vi "GDSString_ParseTextBasedCode.vi"(8 "error in (no error)":errorcluster, 11 "TextIn":string) -> (0 "error out":errorcluster, 3 "Classes":T1[](array[typedef]))   [LabVIEW 2012]
uses:
  <resource>/Framework/Providers/Open_GDS/ClassProviders/Common/String/GDSString_ClassDescriptionType.ctl
  <resource>/Framework/Providers/Open_GDS/ClassProviders/Common/String/GDSString_AccessScopeModifierType.ctl
  <resource>/Framework/Providers/Open_GDS/ClassProviders/Common/String/GDSString_ModifierType.ctl
  <resource>/Framework/Providers/Open_GDS/ClassProviders/Common/String/GDSString_MethodDescriptionType.ctl
  <resource>/Framework/Providers/Open_GDS/ClassProviders/Common/CommonVIs/CommonVIs_AttributeType.ctl
  <resource>/Framework/Providers/Open_GDS/ClassProviders/Common/CommonVIs/CommonVIs_AttributeDataType.ctl
  <resource>/Framework/Providers/Open_GDS/ClassProviders/Common/String/GDSString_ClassParentType.ctl
  <resource>/Framework/Providers/Open_GDS/ClassProviders/Common/String/GDSString_ClassType.ctl
  <resource>/Framework/Providers/Open_GDS/ClassProviders/Common/String/GDSString_ClassOwnerType.ctl
  <resource>/Framework/Providers/Open_GDS/ClassProviders/Common/CommonVIs/CommonVIs_EnumType.ctl
  <resource>/Framework/Providers/Open_GDS/ClassProviders/Common/CommonVIs/CommonVIs_StructType.ctl
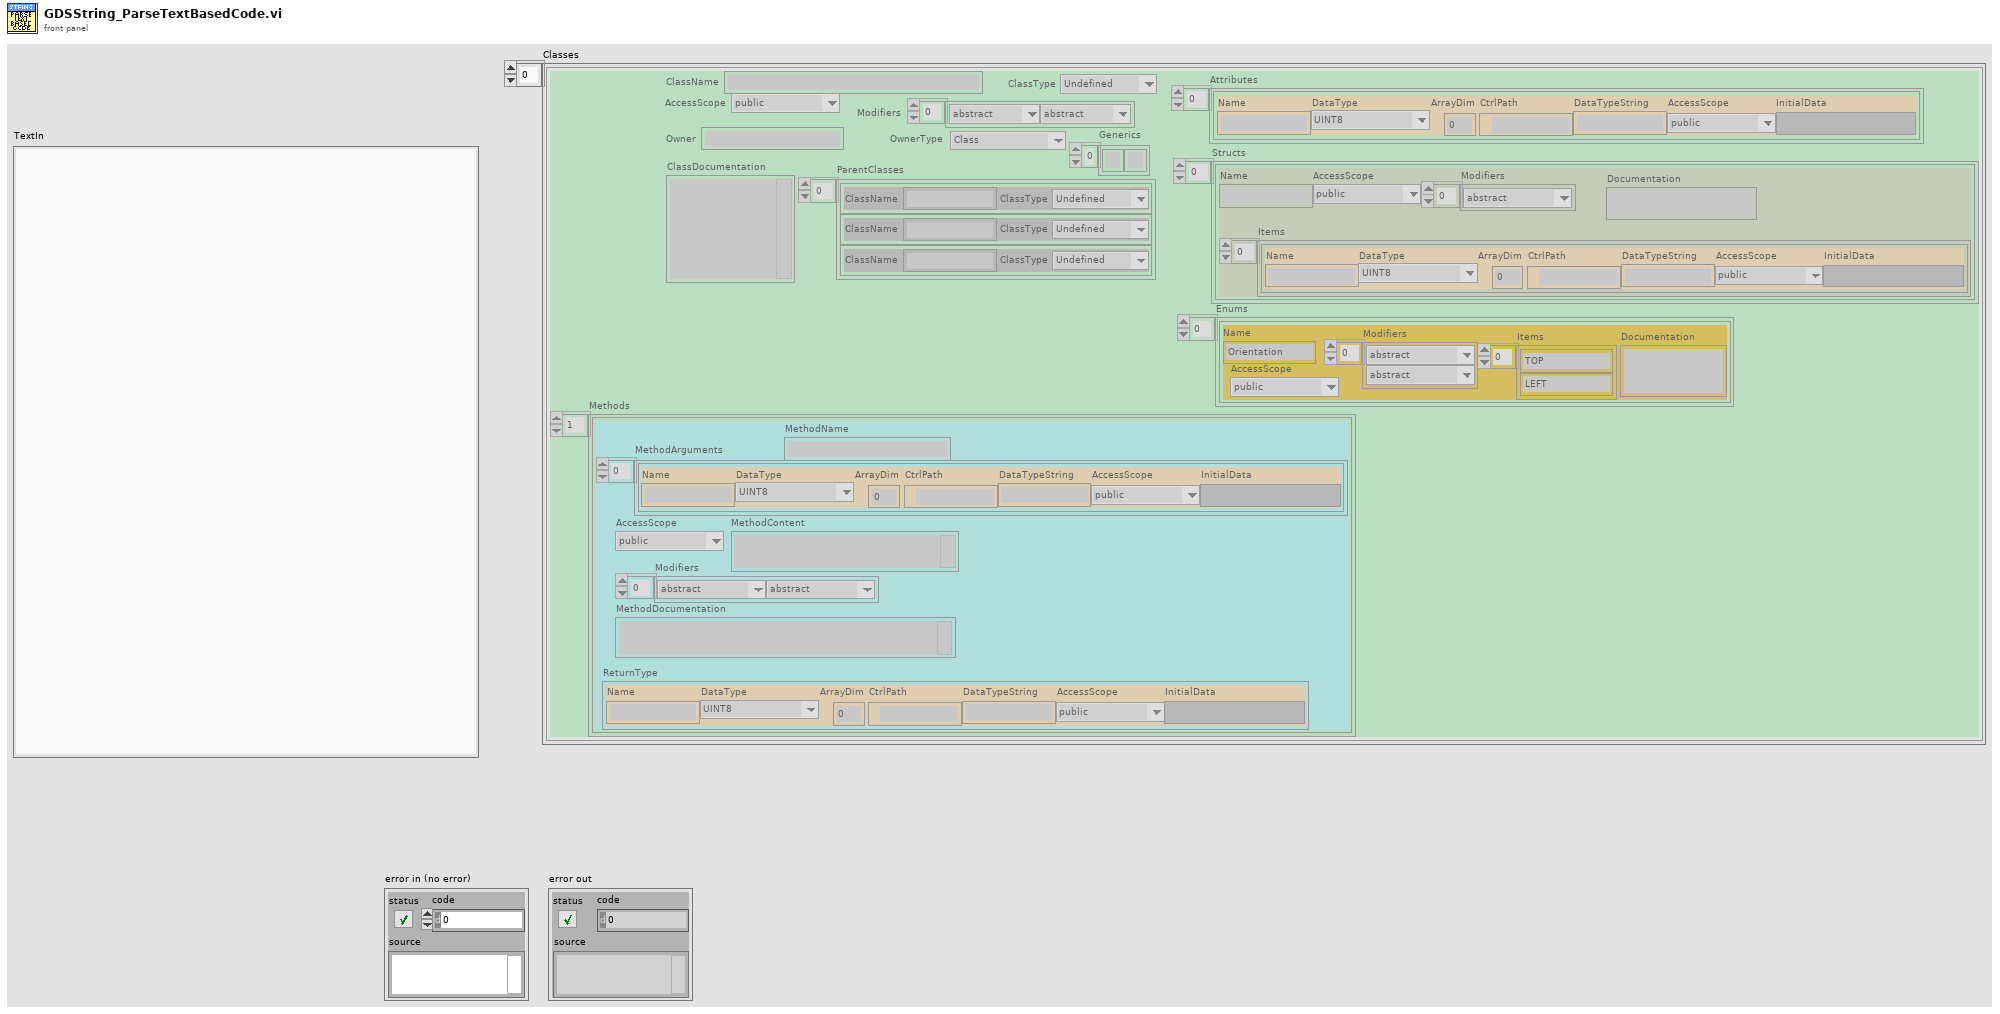
[diagram p1: front panel]
types:
  T1 = typedef "GDSString_ClassDescriptionType.ctl" = cluster{"ClassName":string, "AccessScope":T2, "Modifiers":T3[], "ClassDocumentation":string, "Methods":T4[], "ParentClasses":T7[], "ClassType":T8, "Owner":string, "OwnerType":T9, "Generics":string[], "Attributes":T5[], "Enums":T10[], "Structs":T11[]}
  T2 = typedef "GDSString_AccessScopeModifierType.ctl" = enum16{"public", "private", "protected", "internal"}
  T3 = typedef "GDSString_ModifierType.ctl" = enum16{"abstract", "static", "final", "synchronized", "strictfp", "async", "const", "event", "extern", "new", "override", "partial", "readonly", "sealed", "unsafe", "virtual", "volatile"}
  T4 = typedef "GDSString_MethodDescriptionType.ctl" = cluster{"ReturnType":T5, "MethodName":string, "AccessScope":T2, "Modifiers":T3[], "MethodDocumentation":string, "MethodContent":string, "MethodArguments":T5[]}
  T5 = typedef "CommonVIs_AttributeType.ctl" = cluster{"Name":string, "DataType":T6, "ArrayDim":i32, "CtrlPath":path, "DataTypeString":string, "AccessScope":T2, "InitialData":variant}
  T6 = typedef "CommonVIs_AttributeDataType.ctl" = enum16{"UINT8", "INT8", "UINT16", "INT16", "UINT32", "INT32", "UINT64", "INT64", "SGL", "DBL", "EXT", "CSG", "CDB", "CXT", "TimeStamp", "STRING", "PATH", "BOOL", "ENUM", "RefNum", "VIRefNum", "LabVIEW Class", "Cluster", "Variant", "TypeDef", "Waveform", "LabVIEW Object", "Other", "void"}
  T7 = typedef "GDSString_ClassParentType.ctl" = cluster{"ClassName":string, "ClassType":T8}
  T8 = typedef "GDSString_ClassType.ctl" = enum16{"Undefined", "Class", "Interface"}
  T9 = typedef "GDSString_ClassOwnerType.ctl" = enum16{"NoOwner", "Class", "Package/NameSpace"}
  T10 = typedef "CommonVIs_EnumType.ctl" = cluster{"Name":string, "AccessScope":T2, "Modifiers":T3[], "Items":string[], "Documentation":string}
  T11 = typedef "CommonVIs_StructType.ctl" = cluster{"Name":string, "AccessScope":T2, "Modifiers":T3[], "Items":T5[], "Documentation":string}
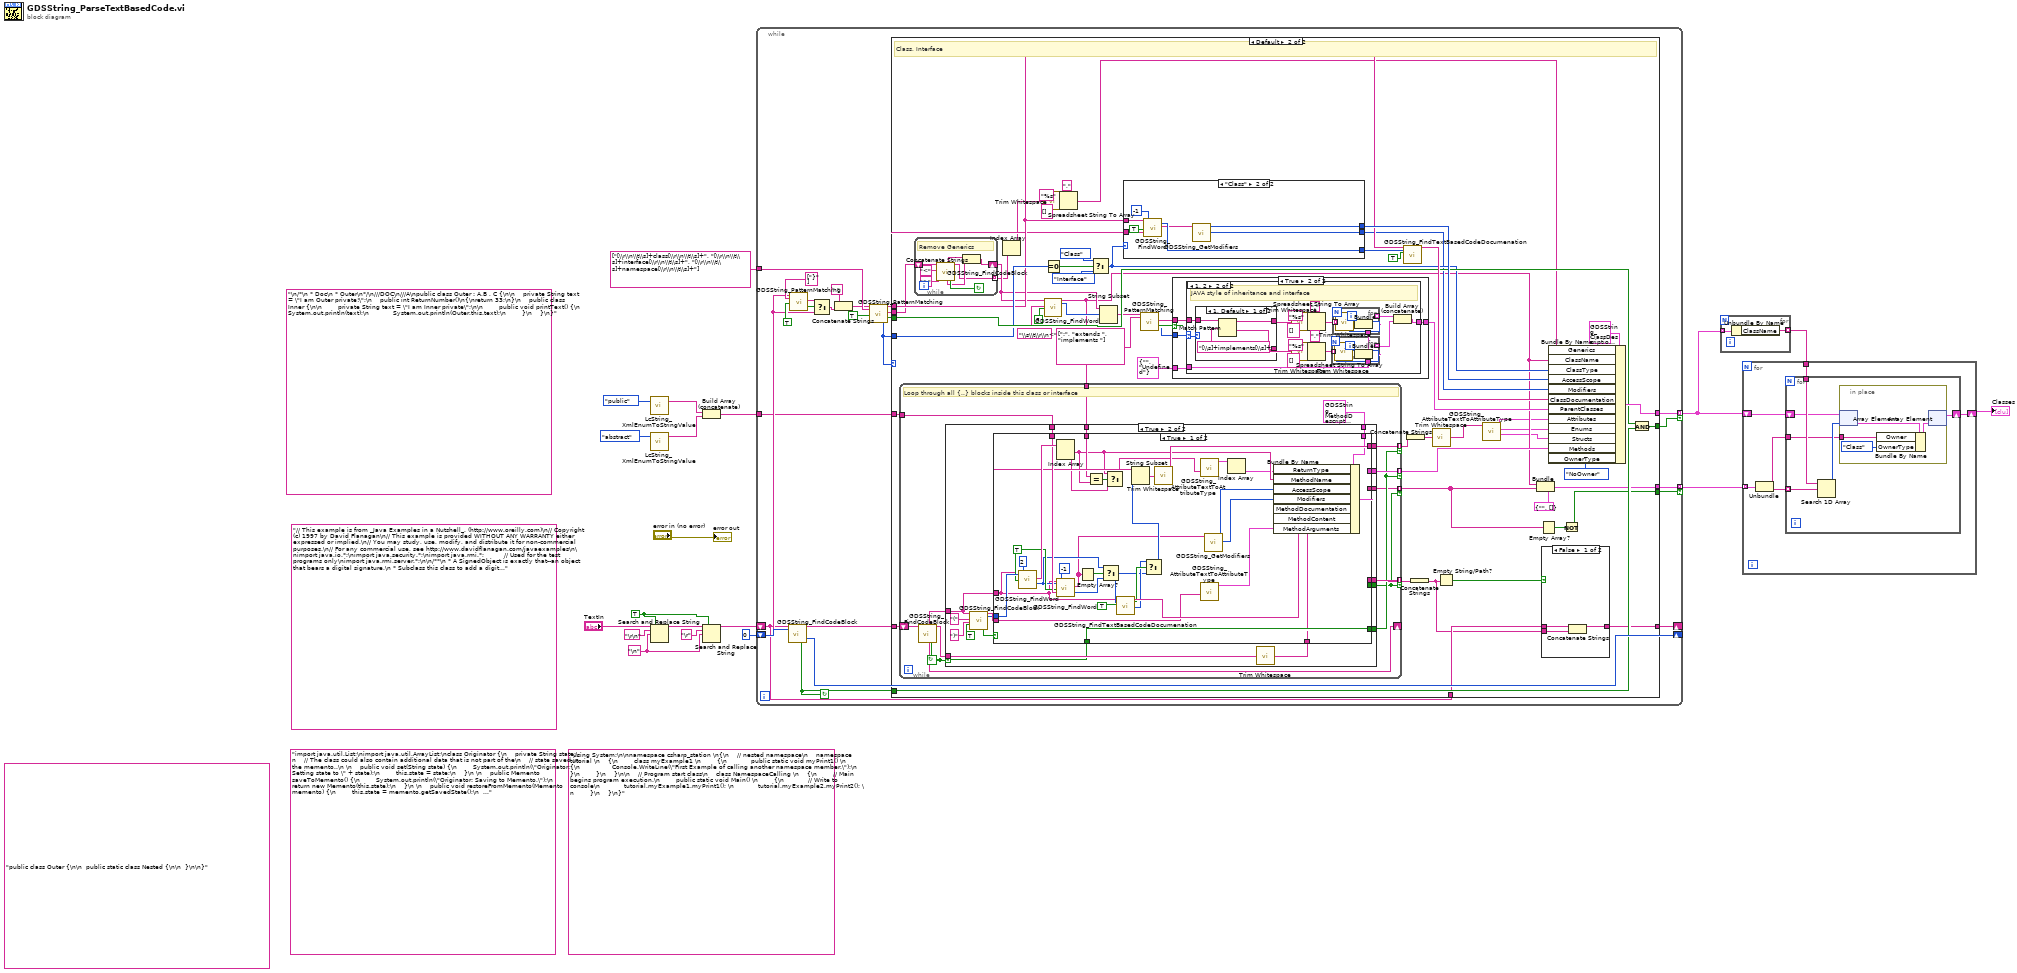
[diagram p0: block diagram]
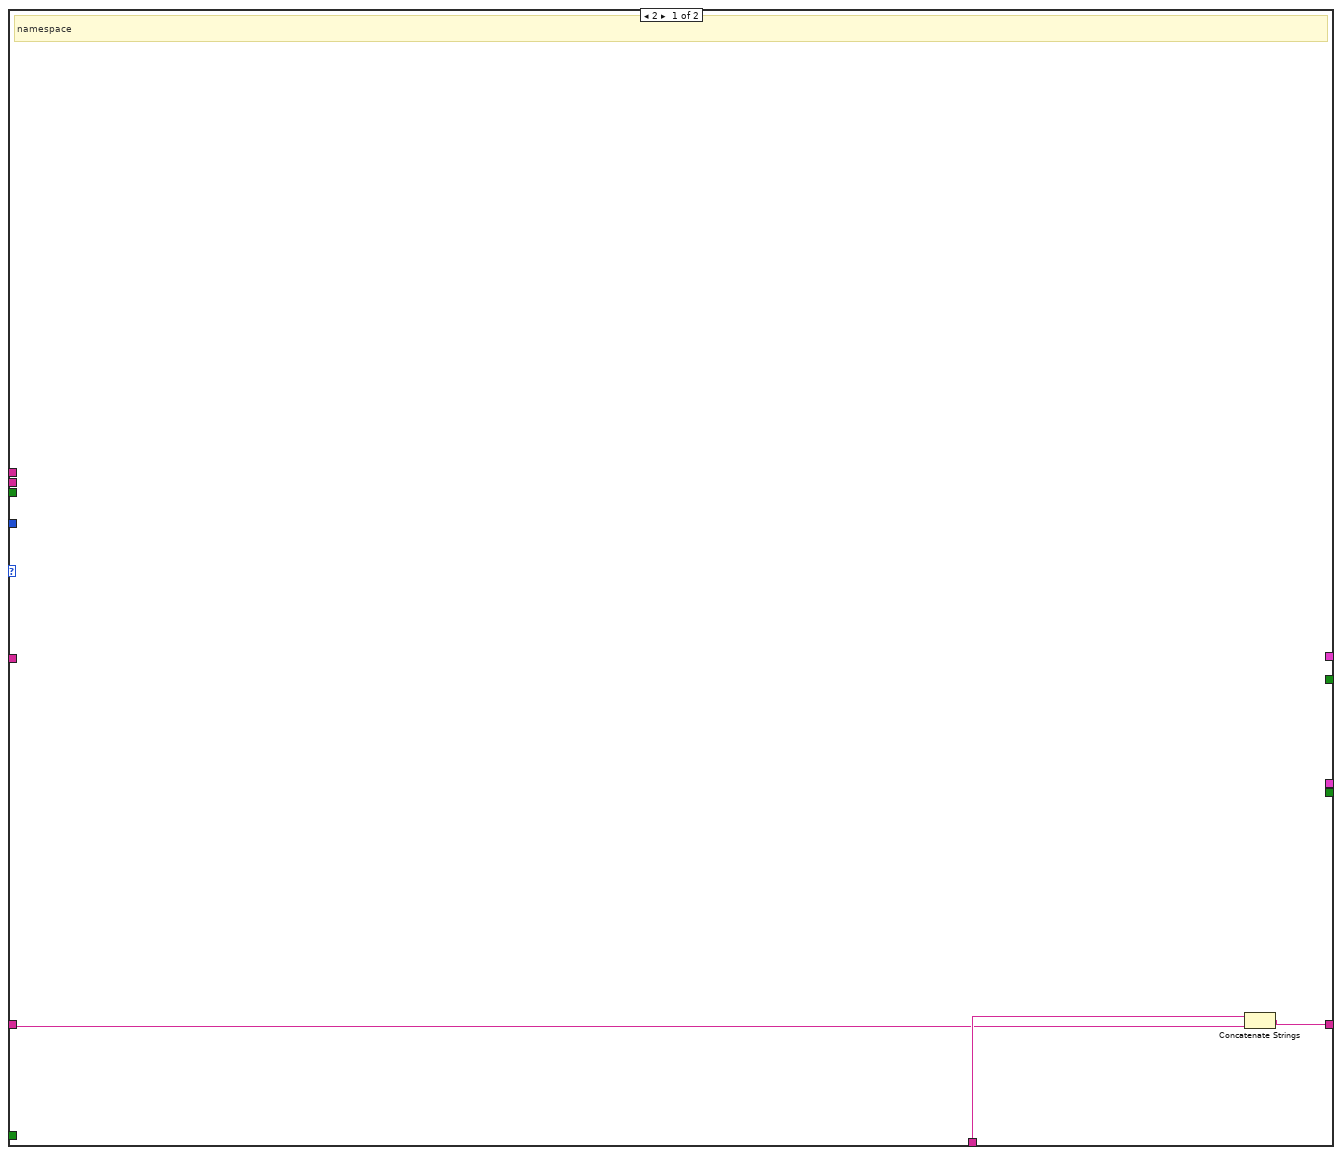
[diagram p2: hidden frame]
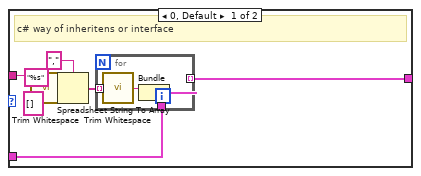
[diagram p5: hidden frame]
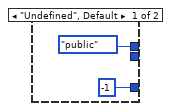
[diagram p7: hidden frame]
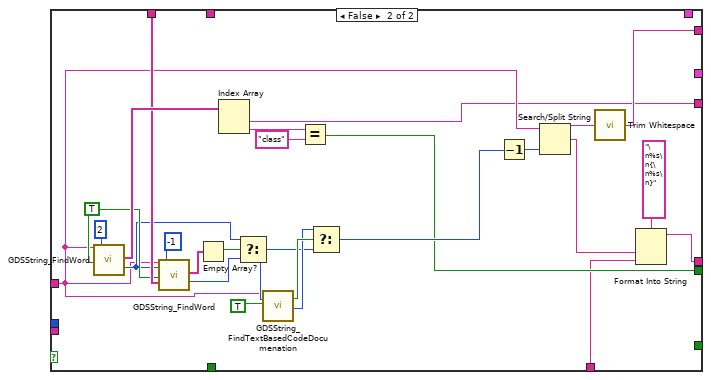
[diagram p9: hidden frame]
diagram:
  (unwired) "using System;\n\nnamespace csharp_station \n{\n    // nested namespace\n    namespace tutorial \n    {\n        class myExample1 \n        {\n            public static void myPrint1() \n            {\n                Console.WriteLine(\"First Example of calling another namespace member.\");\n            }\n        }\n    }\n\n    // Program start class\n    class NamespaceCalling \n    {\n        // Main begins program execution.\n        public static void Main() \n        {\n            // Write to console\n            tutorial.myExample1.myPrint1(); \n            tutorial.myExample2.myPrint2(); \n        }\n    }\n}" ("text")
  (unwired) "public class Outer {\n\n  public static class Nested {\n\n  }\n\n}" ("text")
  (unwired) "import java.util.List;\nimport java.util.ArrayList;\nclass Originator {\n    private String state;\n    // The class could also contain additional data that is not part of the\n    // state saved in the memento..\n \n    public void set(String state) {\n        System.out.println(\"Originator: Setting state to \" + state);\n        this.state = state;\n    }\n \n    public Memento saveToMemento() {\n        System.out.println(\"Originator: Saving to Memento.\");\n        return new Memento(this.state);\n    }\n \n    public void restoreFromMemento(Memento memento) {\n        this.state = memento.getSavedState();\n        System.out.println(\"Originator: State after restoring from Memento: \" + state);\n    }\n \n    public static class Memento {\n        private final String state;\n \n        public Memento(String stateToSave) {\n            state = stateToSave;\n        }\n \n        public String getSavedState() {\n            return state;\n        }\n    }\n}\n \nclass Caretaker {\n    public static void main(String[] args) {\n        List<Originator.Memento> savedStates = new ArrayList<Originator.Memento>();\n \n        Originator originator = new Originator();\n        originator.set(\"State1\");\n        originator.set(\"State2\");\n        savedStates.add(originator.saveToMemento());\n        originator.set(\"State3\");\n        // We can request multiple mementos, and choose which one to roll back to.\n        savedStates.add(originator.saveToMemento());\n        originator.set(\"State4\");\n \n        originator.restoreFromMemento(savedStates.get(1));   \n    }\n}" ("text")
  (unwired) "// This example is from _Java Examples in a Nutshell_. (http://www.oreilly.com)\n// Copyright (c) 1997 by David Flanagan\n// This example is provided WITHOUT ANY WARRANTY either expressed or implied.\n// You may study, use, modify, and distribute it for non-commercial purposes.\n// For any commercial use, see http://www.davidflanagan.com/javaexamples\n\nimport java.io.*;\nimport java.security.*;\nimport java.rmi.*;          // Used for the test programs only\nimport java.rmi.server.*;\n\n/**\n * A SignedObject is exactly that--an object that bears a digital signature.\n * Subclass this class to add a digital signature to any class you want.\n * Note, however, that the signature is computed using serialization, so only\n * the serializable, non-transient fields of a subclass are included in\n * the signature computation.\n **/\npublic class SignedObject implements Serializable {\n  protected String signername;               // Who is doing the signing\n  protected String algorithm;                // What algorithm to use.\n  private byte[] signature;                  // The bytes of the signature\n  transient private boolean signing = false; // A flag used below.\n\n  /**\n   * This method computes a digital signature for the current state of the\n   * object, excluding the signature-related state of this class.\n   * That is, the signature is based only on the state of the subclasses.\n   * The arguments specify who is signing the object, and what digital \n   * signature algorithm to use.\n   * \n   * Note that no other threads should be modifying the object while\n   * this computation is being performed.  If a subclass will be used in a \n   * multi-threaded environment, this means that methods of the subclass\n   * that modify its state should be synchronized like this one is.\n   **/\n  public synchronized void sign(String signername, String algorithm) \n       throws IOException, InvalidKeyException, \n         SignatureException, NoSuchAlgorithmException \n  {\n    // Save the arguments for use by verify()\n    this.signername = signername;\n    this.algorithm = algorithm;\n\n    // Get a Signature object to compute the signature with\n    Signature s = Signature.getInstance(algorithm);\n\n    // Get a Signer object representing the signer\n    Signer signer = \n      (Signer)IdentityScope.getSystemScope().getIdentity(signername);\n\n    // Initialize the Signature object using the PrivateKey of the Signer\n    s.initSign(signer.getPrivateKey());\n\n    // Create an ObjectOutputStream that writes its output to a \n    // ByteArrayStream.  This is how we capture the state of the object\n    // so that it can be signed.\n    ByteArrayOutputStream bout = new ByteArrayOutputStream();\n    ObjectOutputStream out = new ObjectOutputStream(bout);\n\n    // Now serialize the object, capturing its state.  We have to set a flag\n    // before we do this, so that the signer name, algorithm, and signature\n    // itself are not included in this serialized state.  See writeObject()\n    // below to see how this works.\n    signing = true;\n    out.writeObject(this);\n    signing = false;\n\n    // Now tell the Signature object about the bytes of serialized state\n    // that were stored by the ByteArrayOutputStream\n    s.update(bout.toByteArray());\n\n    // And finally, compute the signature\n    this.signature = s.sign();\n  }\n\n  /** A simpler version of sign(), that defaults to using the DSA algorithm */\n  public synchronized void sign(String signername) \n       throws IOException, InvalidKeyException, \n         SignatureException, NoSuchAlgorithmException {\n    sign(signername, \"DSA\");\n  }\n\n  /**\n   * This method verifies the signature of any SignedObject subclass.\n   * It works much like the sign() method, and is also synchronized.\n   **/\n  public synchronized boolean verify() \n       throws IOException, InvalidKeyException,\n         SignatureException, NoSuchAlgorithmException\n  {\n    // Make sure the object is actually signed.\n    if (signature == null) \n      throw new SignatureException(\"Object is not signed\");\n\n    // Get the signature, signer and public key, and initialize, like above,\n    // except that this time use a PublicKey instead of a PrivateKey\n    Signature s = Signature.getInstance(algorithm);\n    Identity signer = \n      (Identity)IdentityScope.getSystemScope().getIdentity(signername);\n    s.initVerify(signer.getPublicKey());\n\n    // Create streams and capture the current state of the object \n    // (excluding the signature bytes themselves) in a byte array\n    ByteArrayOutputStream bout = new ByteArrayOutputStream();\n    ObjectOutputStream out = new ObjectOutputStream(bout);\n    signing = true;\n    out.writeObject(this);\n    signing = false;\n\n    // Pass state of the object to the Signature, and verify the stored\n    // signature bytes against that state.  Return the result of verification.\n    s.update(bout.toByteArray());\n    return s.verify(this.signature);\n  }\n\n  /**\n   * When the contents of the object change, the signature becomes invalid.\n   * When this happens, the signature should be erased, because validation\n   * is guaranteed to fail.\n   **/\n  public void removeSignature() { \n    signature = null; signername = null; algorithm = null; \n  }\n\n  /**\n   * This method is invoked to allow custom serialization.\n   * We only write out our signature-related state when we are not computing\n   * or verifying a signature.  When we are computing or verifying, only our\n   * subclass state gets written out.  If we don't do this, verification will\n   * fail because the signature[] array will obviously be different on\n   * verification than it is when the signature is generated.\n   **/\n  private void writeObject(ObjectOutputStream out) throws IOException {\n    if (!signing) out.defaultWriteObject();\n  }\n}\n\n/**\n * This class is a simple SignedObject subclass.\n * This and the following interface and classes are used to test SignedObject.\n **/\nclass SignedString extends SignedObject {\n  public String s;\n  public SignedString(String s) { this.s = s; }\n}\n\n/**\n * This interface extends Remote.  It is part of an RMI example using our\n * SignedString class above.\n **/\ninterface RemoteSignedString extends Remote {\n  public SignedString getString() throws RemoteException;\n}\n\n/**\n * This is a simple RMI server class and a program to start and register the\n * server.  The server creates a SignedString object, signs it, and then \n * exports it to clients through the RemoteSignedString getString() method.\n **/\nclass SignedStringServer extends UnicastRemoteObject \n                         implements RemoteSignedString \n{\n  SignedString s;  // The state of the server object\n\n  /** The constructor.  Initialize the SignedString */\n  public SignedStringServer(SignedString s) throws RemoteException {this.s=s;}\n\n  /** This is the remote method exported by the server */\n  public SignedString getString() throws RemoteException { return s; }\n  \n  /** The main program that creates and registers the server object */\n  public static void main(String[] args) \n       throws NoSuchAlgorithmException, InvalidKeyException, \n         IOException, SignatureException\n  {\n    SignedString ss = new SignedString(args[0]);         // create object\n    ss.sign(args[1]);                                    // sign it\n    SignedStringServer sss = new SignedStringServer(ss); // start server\n    Naming.rebind(\"SignedStringServer\", sss);            // register server\n    System.out.println(\"Ready for clients\");             // up and running!\n  }\n}\n\n/**\n * This class is a client that connects to a RemoteSignedString server and\n * calls the getString() method to obtain a SignedString.  It then verifies\n * the signature of the object that it has just downloaded over a network\n * from an entirely different Java VM.  The client takes an optional hostname\n * argument on the command line.\n **/\nclass SignedStringClient {\n  public static void main(String[] args)\n       throws NoSuchAlgorithmException, InvalidKeyException, \n         IOException, SignatureException, NotBoundException\n  {\n    // Look up the server\n    RemoteSignedString rss = \n      (RemoteSignedString) Naming.lookup(\"rmi://\" + \n                                         ((args.length>0)?args[0]:\"\") +\n                                         \"/SignedStringServer\"); \n\n    // Invoke a remote method of the server to get a SignedString\n    SignedString ss = rss.getString();\n\n    // Now verify the signature on that SignedString.\n    if (ss.verify()) System.out.println(\"Verified SignedString: \" + ss.s);\n    else System.out.println(\"SignedString failed verification\");\n  }\n}\n" ("text")
  w14 = TRUE ("replace all? (F)")
  w12 = "\n" ("search string")
  (unwired) "\n/*\n * Doc\n * Outer\n*/\n///DOC\n///A\npublic class Outer : A,B , C {\n\n    private String text = \"I am Outer private!\";\n    public int ReturnNumber()\n{\nreturn 33;\n}\n    public class Inner {\n\n        private String text = \"I am Inner private\";\n\n        public void printText() {\n            System.out.println(text);\n            System.out.println(Outer.this.text);\n        }\n    }\n}" ("text")
  n1 = call <userlib>:"LcString_XmlEnumToStringValue.vi"("EnumVariantIn(used if String is Empty)"=GDSString_AccessScopeModifierType."public" ("AccessScope")) -> ("EnumItems(string)"=w1:string[])  [unwired: 15 in, 3 out]
  n2 = call <userlib>:"LcString_XmlEnumToStringValue.vi"("EnumVariantIn(used if String is Empty)"=GDSString_ModifierType."abstract" ("Modifiers")) -> ("EnumItems(string)"=w2:string[])  [unwired: 15 in, 3 out]
  n3 = Search and Replace String(replace all?=w14, input string="TextIn", search string="\r\n", replace string=w12) -> (result string=w16:string)  [unwired: 4 in, 3 out]
  n4 = Build Array (concatenate)(w1, w2) -> (w17:string[])
  n5 = Search and Replace String(replace all?=w14, input string=w16, search string="\r", replace string=w12) -> (result string=w11:string)  [unwired: 4 in, 3 out]
  n6 = while {
    tunnel: w17 -> [w28]
    shift-right: [w42] -> _
    shift-left: 0 ("GetNext-X_Words(1,-1=All)") -> [w43]
    tunnel: [w41] -> w8 mode=indexing if=w32
    shift-right: [w26] -> _
    shift-left: w11 -> [w27]
    tunnel: [w25] -> w9 mode=indexing if=w24
    tunnel: string[] ["[\\r\\n\\t\\s]+class[\\r\\n\\t\\s]+", "[\\r\\n\\t\\s]+interface[\\r\\n\\t\\s]+", "[\\r\\n\\t\\s]+namespace[\\r\\n\\t\\s]+"] -> [w23]
    stop <- w33 continue-if-true
    n7 = call <resource>:"GDSString_FindCodeBlock.vi"("Text"=w27, "StringStartOffset(Default=-1 => 0 for Forward, StrLenght for Backwards)"=w43) -> ("TextBeforeBlock"=w35:string, "found"=w33:bool, "BlockText"=w44:string, "BlockEnd(Outside)"=w42:i32)  [unwired: 9 in, 5 out]
    n8 = call <resource>:"GDSString_PatternMatching.vi"("TextIn"=w35, "PatternMatchingStrings"=string[] ["}"] ("PatternMatchingString"), "Search Backwards"=TRUE) -> ("TextAfter"=w36:string, "Found"=w37:bool)  [unwired: 10 in, 5 out]
    n9 = Select(t=w36, s=w37, f=w35) -> (s? t:f=w34:string)
    n10 = Concatenate Strings(" " ("string"), w34) -> (w21:string)
    n11 = call <resource>:"GDSString_PatternMatching.vi"("TextIn"=w21, "PatternMatchingStrings"=w23, "Search Backwards"=TRUE) -> ("IndexOfTheFoundPatternMatchingString"=w22:i32, "TextBefore"=w29:string, "TextAfter"=w30:string, "Found"=w31:bool)  [unwired: 10 in, 3 out]
    n12 = case shown="Default" w22 {
      tunnel: w44 -> [w46 w103]
      tunnel: [_ w100] -> w41
      tunnel: w33 -> [_ w95]
      tunnel: [_ w94] -> w32
      tunnel: w31 -> [_ w93]
      tunnel: w22 -> [_ w92]
      tunnel: w30 -> [_ w62]
      tunnel: w29 -> [_ w87]
      tunnel: w28 -> [_ w80]
      tunnel: w27 -> [w47 w73]
      tunnel: [w45 w70] -> w26
      tunnel: [_ w68] -> w25
      tunnel: [_ w53] -> w24
      frame 2 {
        # "namespace"
        n13 = Concatenate Strings(w47, w46) -> (w45:string)
      }
      frame Default {
        # "Class, Interface"
        n14 = while {
          shift-right: [w105] -> w61
          shift-left: w62 -> [w111]
          tunnel: [w104] -> w60 mode=indexing
          stop <- w108 continue-if-true
          # "Remove Generics"
          n15 = call <resource>:"GDSString_FindCodeBlock.vi"("Text"=w111, "CodeBlockStartCharacter( { )"="<", "CodeBlockEndCharacter( } )"=">") -> ("TextBeforeBlock"=w107:string, "TextAfterBlock"=w106:string, "found"=w108:bool, "BlockText"=w104:string)  [unwired: 8 in, 5 out]
          n16 = Concatenate Strings(w107, w106) -> (w105:string)
        }
        n17 = Index Array(array=w60) -> (element=w56:string)  [unwired: 1 in]
        n18 = call <vilib>:"Trim Whitespace.vi"("string"=w56) -> ("trimmed string"=w59:string)  [unwired: 1 in]
        n19 = call <resource>:"GDSString_FindWord.vi"("Text"=w61, "PatternMatchingDelimiter(\\s\\t\\r\\n)"="\\s\\t\\r\\n<" ("PatternMatchingDelimiter(\\s\\t\\r\\n)"), "Search Backwards"=FALSE) -> ("NextWord"=w52:string, "IndexAfterMatch(Or before when searching Backwards)"=w88:i32)  [unwired: 11 in, 4 out]
        n20 = while {
          shift-right: [w187] -> _
          shift-left: w103 -> [w188]
          tunnel: [w186] -> w98 mode=indexing if=w180
          tunnel: [w185] -> w99 mode=indexing if=w180
          tunnel: w80 -> [w184]
          tunnel: [w181] -> w72 mode=indexing if=w178
          tunnel: [w179] -> w67 mode=indexing if=w178
          tunnel: w52 -> [w175]
          stop <- w177 continue-if-true
          # "Loop through all {..} blocks inside this class or interface"
          n21 = call <resource>:"GDSString_FindCodeBlock.vi"("Text"=w188) -> ("TextBeforeBlock"=w182:string, "TextAfterBlock"=w187:string, "found"=w177:bool, "BlockText"=w183:string)  [unwired: 10 in, 5 out]
          n22 = case shown="True" w177 {
            selector: w177 -> [_ w191]
            tunnel: [_ w207] -> w186
            tunnel: [_ w203] -> w185
            tunnel: T4 {"ReturnType"={"Name"="", "DataType"=enum."UINT8", "ArrayDim"=0, "CtrlPath"=path "", "DataTypeString"="", "AccessScope"=enum."public", "InitialData"=variant}, "MethodName"="", "AccessScope"=enum."public", "Modifiers"=[], "MethodDocumentation"="", "MethodContent"="", "MethodArguments"=[]} -> [_ w201]
            tunnel: w184 -> [_ w200]
            tunnel: w183 -> [_ w199]
            tunnel: w182 -> [_ w197]
            tunnel: [_ w195] -> w181
            tunnel: [_ w194] -> w180
            tunnel: [_ w193] -> w179
            tunnel: [_ w192] -> w178
            tunnel: w175 -> [_ w189]
            frame False {
            }
            frame True {
              n23 = call <resource>:"GDSString_FindCodeBlock.vi"("Text"=w197, "CodeBlockStartCharacter( { )"="(", "CodeBlockEndCharacter( } )"=")", "Search Backwards"=TRUE) -> ("found"=w196:bool, "BlockText"=w202:string, "BlockStart(Outside)"=w198:i32)  [unwired: 7 in, 6 out]
              n24 = call <vilib>:"Trim Whitespace.vi"("string"=w199) -> ("trimmed string"=w190:string)  [unwired: 1 in]
              n25 = case shown="True" w196 {
                tunnel: [w241 w254] -> w207
                tunnel: [w240 _] -> w203
                tunnel: w202 -> [w209 _]
                tunnel: w201 -> [w238 _]
                tunnel: w200 -> [w235 w265]
                tunnel: w190 -> [w219 w243]
                tunnel: w198 -> [w232 _]
                tunnel: w197 -> [w221 w251]
                tunnel: [_ w242] -> w195
                tunnel: w191 -> [w220 _]
                tunnel: [w220 _] -> w194
                tunnel: [_ w247] -> w192
                tunnel: [_ w246] -> w193
                tunnel: w189 -> [w217 _]
                frame True {
                  w229 = TRUE ("Search Backwards")
                  n26 = call <resource>:"GDSString_FindWord.vi"("Text"=w221, "StringStartOffset(Default=-1 => 0 for Forward, StrLenght for Backwards)"=w232, "Search Backwards"=w229, "GetNext-X_Words(1,-1=All)"=2 ("GetNext-X_Words(1)")) -> ("NextWords"=w239:string[], "IndexAfterLastMatch(Or before when searching Backwards)"=w223:i32)  [unwired: 10 in, 4 out]
                  n27 = call <resource>:"GDSString_FindWord.vi"("Text"=w221, "StringStartOffset(Default=-1 => 0 for Forward, StrLenght for Backwards)"=w223, "Search Backwards"=w229, "AllowedWords(PatternMatching)"=w235, "GetNext-X_Words(1,-1=All)"=-1) -> ("NextWords"=w213:string[], "IndexAfterLastMatch(Or before when searching Backwards)"=w227:i32)  [unwired: 9 in, 4 out]
                  n28 = Index Array(array=w239) -> (element #1=w215:string, element #2=w214:string)  [unwired: 2 in]
                  n29 = Empty Array?(array=w213) -> (empty?=w228:bool)
                  n30 = Equal?(x=w217, y=w215) -> (x = y?=w216:bool)
                  n31 = Select(t=w223, s=w228, f=w227) -> (s? t:f=w222:i32)
                  n32 = Select(t=w215, s=w216, f=w214) -> (s? t:f=w212:string)
                  n33 = call <resource>:"GDSString_FindTextBasedCodeDocumenation.vi"("Text"=w221, "StringStartOffset(Default=-1 => 0 for Forward, StrLenght for Backwards)"=w222, "Search Backwards"=TRUE) -> ("Document"=w234:string, "Found"=w226:bool, "IndexBeforeDocument(Or after when searching Backwards)"=w225:i32)  [unwired: 12 in, 2 out]
                  n34 = Select(t=w225, s=w226, f=w222) -> (s? t:f=w224:i32)
                  n35 = String Subset(string=w221, length (rest)=w224) -> (substring=w231:string)  [unwired: 1 in]
                  n36 = call <vilib>:"Trim Whitespace.vi"("string"=w231) -> ("trimmed string"=w241:string)  [unwired: 1 in]
                  n37 = call <resource>:"GDSString_AttributeTextToAttributeType.vi"("MethodText"=w212) -> ("Attributes"=w211:T5[])  [unwired: 7 in, 3 out]
                  n38 = call <resource>:"GDSString_AttributeTextToAttributeType.vi"("MethodText"=w209) -> ("Attributes"=w208:T5[])  [unwired: 7 in, 3 out]
                  n39 = call <resource>:"GDSString_GetModifiers.vi"("Words"=w213) -> ("Array out"=w237:T3[], "AccessScope"=w218:T2)  [unwired: 8 in, 1 out]
                  n40 = Index Array(array=w211) -> (element=w210:T5)  [unwired: 1 in]
                  n41 = Bundle By Name(cluster=w238, "ReturnType"=w210, "MethodName"=w215, "AccessScope"=w218, "Modifiers"=w237, "MethodDocumentation"=w234, "MethodContent"=w219, "MethodArguments"=w208) -> (w240:T4)
                }
                frame False {
                  w261 = TRUE ("Search Backwards")
                  n42 = call <resource>:"GDSString_FindWord.vi"("Text"=w251, "Search Backwards"=w261, "GetNext-X_Words(1,-1=All)"=2 ("GetNext-X_Words(1)")) -> ("NextWords"=w267:string[], "IndexAfterLastMatch(Or before when searching Backwards)"=w256:i32)  [unwired: 11 in, 4 out]
                  n43 = call <resource>:"GDSString_FindWord.vi"("Text"=w251, "StringStartOffset(Default=-1 => 0 for Forward, StrLenght for Backwards)"=w256, "Search Backwards"=w261, "AllowedWords(PatternMatching)"=w265, "GetNext-X_Words(1,-1=All)"=-1) -> ("NextWords"=w263:string[], "IndexAfterLastMatch(Or before when searching Backwards)"=w259:i32)  [unwired: 9 in, 4 out]
                  n44 = Empty Array?(array=w263) -> (empty?=w260:bool)
                  n45 = Index Array(array=w267) -> (element #1=w246:string, element #2=w253:string)  [unwired: 2 in]
                  n46 = Select(t=w256, s=w260, f=w259) -> (s? t:f=w255:i32)
                  n47 = call <resource>:"GDSString_FindTextBasedCodeDocumenation.vi"("Text"=w251, "StringStartOffset(Default=-1 => 0 for Forward, StrLenght for Backwards)"=w255, "Search Backwards"=TRUE) -> ("Found"=w258:bool, "IndexBeforeDocument(Or after when searching Backwards)"=w257:i32)  [unwired: 12 in, 3 out]
                  n48 = Equal?(x=w253, y="class") -> (x = y?=w247:bool)
                  n49 = Select(t=w257, s=w258, f=w255) -> (s? t:f=w250:i32)
                  n50 = Decrement(x=w250) -> (x-1=w249:i32)
                  n51 = Search/Split String(string=w251, offset (0)=w249) -> (substring before match=w248:string, match + rest of string=w244:string)  [unwired: 1 in, 1 out]
                  n52 = call <vilib>:"Trim Whitespace.vi"("string"=w248) -> ("trimmed string"=w254:string)  [unwired: 1 in]
                  n53 = Format Into String(format string="\n%s\n{\n%s\n}", w244, w243) -> (resulting string=w242:string)  [unwired: 2 in, 1 out]
                }
              }
            }
          }
        }
        n54 = Equal To 0?(x=w92) -> (x = 0?=w91:bool)
        n55 = Spreadsheet String To Array(delimiter (Tab)=",", format string="%s", spreadsheet string=w59, array type (2D Dbl)=string[] [] ("PatternMatchingString")) -> (array=w54:string[])
        n56 = Select(t=GDSString_ClassType."Class" ("ClassType"), s=w91, f=GDSString_ClassType."Interface" ("ClassType")) -> (s? t:f=w85:T8)
        n57 = String Subset(string=w61, offset (0)=w88) -> (substring=w84:string)  [unwired: 1 in]
        n58 = case shown="\"Class\"" w85 {
          tunnel: [GDSString_AccessScopeModifierType."public" ("AccessScope") w168] -> w101
          tunnel: w80 -> [_ w173]
          tunnel: w87 -> [_ w172]
          tunnel: [-1 ("IndexAfterMatch(Or before when searching Backwards)") w171] -> w86
          tunnel: [_ w167] -> w78
          frame "Undefined", Default {
          }
          frame "Class" {
            n59 = call <resource>:"GDSString_FindWord.vi"("Text"=w172, "Search Backwards"=TRUE, "AllowedWords(PatternMatching)"=w173, "GetNext-X_Words(1,-1=All)"=-1) -> ("IndexAfterMatch(Or before when searching Backwards)"=w171:i32, "NextWords"=w169:string[])  [unwired: 10 in, 4 out]
            n60 = call <resource>:"GDSString_GetModifiers.vi"("Words"=w169) -> ("Array out"=w167:T3[], "AccessScope"=w168:T2)  [unwired: 8 in, 1 out]
          }
        }
        n61 = call <resource>:"GDSString_PatternMatching.vi"("TextIn"=w84, "PatternMatchingStrings"=string[] [":", "extends ", "implements "]) -> ("IndexOfTheFoundPatternMatchingString"=w81:i32, "TextAfter"=w77:string, "Found"=w82:bool)  [unwired: 11 in, 4 out]
        n62 = case shown="True" w82 {
          tunnel: w81 -> [_ w119]
          tunnel: w77 -> [_ w118]
          tunnel: T7 {"ClassName"="", "ClassType"=enum."Undefined"} ("Parent") -> [_ w117]
          tunnel: [_ w116] -> w75
          frame False {
          }
          frame True {
            n63 = case shown="1, 2" w119 {
              selector: w119 -> [_ w148]
              tunnel: w118 -> [w127 w149]
              tunnel: w117 -> [w120 w134]
              tunnel: [w121 w140] -> w116
              frame 0, Default {
                # "c# way of inheritens or interface"
                n64 = call <vilib>:"Trim Whitespace.vi"("string"=w127) -> ("trimmed string"=w124:string)  [unwired: 1 in]
                n65 = Spreadsheet String To Array(delimiter (Tab)=",", format string="%s", spreadsheet string=w124, array type (2D Dbl)=string[] [] ("PatternMatchingString")) -> (array=w123:string[])
                n66 = for {
                  tunnel: w123 -> [w130] mode=indexing
                  tunnel: w120 -> [w131]
                  tunnel: [w129] -> w121 mode=indexing
                  n67 = call <vilib>:"Trim Whitespace.vi"("string"=w130) -> ("trimmed string"=w128:string)  [unwired: 1 in]
                  n68 = Bundle(cluster=w131, "ClassName"=w128) -> (w129:T7)  [unwired: 1 in]
                }
              }
              frame 1, 2 {
                # "JAVA style of inheritance and interface"
                n69 = case shown="1, Default" w148 {
                  tunnel: w149 -> [w163 w164]
                  tunnel: [w161 _] -> w142
                  tunnel: [w160 w164] -> w132
                  frame 1, Default {
                    n70 = Match Pattern(string=w163, regular expression="[\\s]+implements[\\s]+") -> (before substring=w161:string, after substring=w160:string)  [unwired: 1 in, 2 out]
                  }
                  frame 2 {
                  }
                }
                n71 = call <vilib>:"Trim Whitespace.vi"("string"=w142) -> ("trimmed string"=w145:string)  [unwired: 1 in]
                n72 = call <vilib>:"Trim Whitespace.vi"("string"=w132) -> ("trimmed string"=w137:string)  [unwired: 1 in]
                n73 = Spreadsheet String To Array(delimiter (Tab)=",", format string="%s", spreadsheet string=w145, array type (2D Dbl)=string[] [] ("PatternMatchingString")) -> (array=w144:string[])
                n74 = Spreadsheet String To Array(delimiter (Tab)=",", format string="%s", spreadsheet string=w137, array type (2D Dbl)=string[] [] ("PatternMatchingString")) -> (array=w138:string[])
                n75 = for {
                  tunnel: w138 -> [w153] mode=indexing
                  tunnel: w134 -> [w154]
                  tunnel: [w152] -> w133 mode=indexing
                  n76 = call <vilib>:"Trim Whitespace.vi"("string"=w153) -> ("trimmed string"=w151:string)  [unwired: 1 in]
                  n77 = Bundle(cluster=w154, "ClassName"=w151, "ClassType"=GDSString_ClassType."Interface") -> (w152:T7)
                }
                n78 = for {
                  tunnel: w144 -> [w158] mode=indexing
                  tunnel: w134 -> [w159]
                  tunnel: [w157] -> w141 mode=indexing
                  n79 = call <vilib>:"Trim Whitespace.vi"("string"=w158) -> ("trimmed string"=w156:string)  [unwired: 1 in]
                  n80 = Bundle(cluster=w159, "ClassName"=w156, "ClassType"=GDSString_ClassType."Class") -> (w157:T7)
                }
                n81 = Build Array (concatenate)(w141, w133) -> (w140:T7[])
              }
            }
          }
        }
        n82 = call <resource>:"GDSString_FindTextBasedCodeDocumenation.vi"("Text"=w87, "StringStartOffset(Default=-1 => 0 for Forward, StrLenght for Backwards)"=w86, "Search Backwards"=TRUE) -> ("Document"=w96:string)  [unwired: 12 in, 4 out]
        n83 = Concatenate Strings(w98) -> (w74:string)
        n84 = Concatenate Strings(w72) -> (w69:string)
        n85 = call <vilib>:"Trim Whitespace.vi"("string"=w74) -> ("trimmed string"=w51:string)  [unwired: 1 in]
        n86 = Empty String/Path?(string/path=w69) -> (empty?=w71:bool)
        n87 = call <resource>:"GDSString_AttributeTextToAttributeType.vi"("AttributeText"=w51) -> ("Structs"=w48:T11[], "Enums"=w49:T10[], "Attributes"=w50:T5[])  [unwired: 7 in, 1 out]
        n88 = Bundle(cluster=cluster{"Owner":string, "Nested":string[]} {"Owner"="", "Nested"=[]}, "Owner"=w52, "Nested"=w67) -> (w68:cluster{"Owner":string, "Nested":string[]})
        n89 = Empty Array?(array=w67) -> (empty?=w66:bool)
        n90 = case shown="False" w71 {
          tunnel: w73 -> [w114 w115]
          tunnel: [w113 w115] -> w70
          tunnel: w69 -> [w112 _]
          frame False {
            n91 = Concatenate Strings(w114, w112) -> (w113:string)
          }
          frame True {
          }
        }
        n92 = Bundle By Name(cluster=T1 {"ClassName"="", "AccessScope"=enum."public", "Modifiers"=[], "ClassDocumentation"="", "Methods"=[], "ParentClasses"=[], "ClassType"=enum."Undefined", "Owner"="", "OwnerType"=enum."NoOwner", "Generics"=[], "Attributes"=[], "Enums"=[], "Structs"=[]} ("Class"), "Generics"=w54, "ClassName"=w52, "ClassType"=w85, "AccessScope"=w101, "Modifiers"=w78, "ClassDocumentation"=w96, "ParentClasses"=w75, "Attributes"=w50, "Enums"=w49, "Structs"=w48, "Methods"=w99, "OwnerType"=GDSString_ClassOwnerType."NoOwner") -> (w100:T1)
        n93 = Not(x=w66) -> (.not. x?=w53:bool)
        n94 = And(x=w93, y=w95) -> (x .and. y?=w94:bool)
      }
    }
  }
  n95 = for {
    tunnel: w8 -> [w269] mode=indexing
    tunnel: [w268] -> w7 mode=indexing
    n96 = Unbundle By Name(w269) -> ("ClassName"=w268:string)
  }
  n97 = for {
    tunnel: w9 -> [w275] mode=indexing
    shift-right: [w270] -> w6
    shift-left: w8 -> [w273]
    tunnel: w7 -> [w272]
    n98 = Unbundle(w275) -> ("Owner"=w271:string, "Nested"=w274:string[])
    n99 = for {
      tunnel: w274 -> [w281] mode=indexing
      shift-right: [w276] -> w270
      shift-left: w273 -> [w279]
      tunnel: w272 -> [w280]
      tunnel: w271 -> [w277]
      n100 = Search 1D Array(1D array=w280, element=w281) -> (index of element=w278:i32)  [unwired: 1 in]
      n101 = in-place {
        in-place-border: w277 -> [w283]
        n102 = in-place-array #1(w279, w278) -> (w285:T1)
        n103 = Bundle By Name(cluster=w285, "Owner"=w283, "OwnerType"=GDSString_ClassOwnerType."Class") -> (w284:T1)
        n104 = in-place-array #1(w284) -> (w276:T1[])  [unwired: 1 out]
      }
    }
  }
  "Classes" <- w6
  "error out" <- "error in (no error)"
